vi "ASI Pulse Guide Off.vi"(10 "direction":i32, 11 "iCameraID":i32) -> (3 "function return":i32)   [LabVIEW 2023, in "ASICamera2_no_err.lvlib"]
doc: "ASICAMERA_API ASI_ERROR_CODE ASIPulseGuideOff(int iCameraID, ASI_GUIDE_DIRECTION direction);"
uses:
  ASICamera2_no_err.lvlib
  ASICamera2.dll
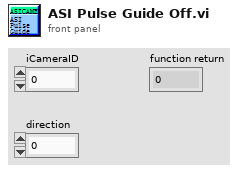
[diagram p1: front panel]
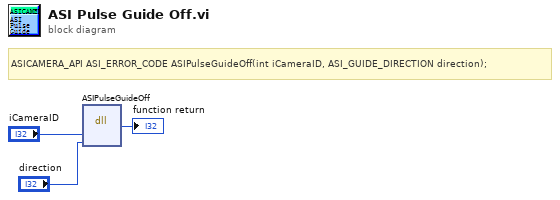
[diagram p0: block diagram]
diagram:
  # "ASICAMERA_API ASI_ERROR_CODE ASIPulseGuideOff(int iCameraID, ASI_GUIDE_DIRECTION direction);"
  n1 = dll-call lib="C:/Users/quantum/Documents/LVDAQ/ConcreteClasses/ConcreteInstrumentClasses/CameraClasses/ZWO_ASI_LV/Labview_ASI_demo_64bit_221128/user.lib/ASICamera2_no_err/ASICamera2.*" fn="ASIPulseGuideOff"("iCameraID"="iCameraID", "direction"="direction") -> (→"function return":i32)  [unwired: 5 in, 2 out]
